vi "Configure Multicolumn Listbox for Displayed Samples.vi"(7 "Samples":i64, 8 "error in":errorcluster, 11 "MulticolumnListbox in":refnum<vi>) -> (0 "error out":errorcluster, 3 "MulticolumnListbox out":refnum<vi>)   [LabVIEW 2018, in "NI_TDMS File Viewer.lvlib"]
uses:
  NI_TDMS File Viewer.lvlib
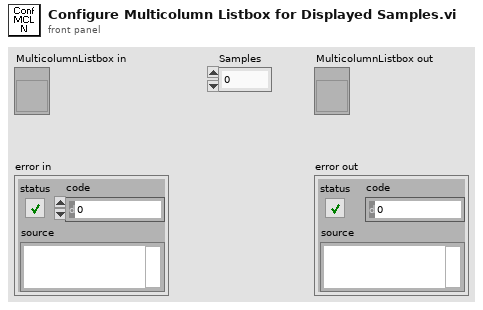
[diagram p1: front panel]
types:
  T1 = typedef "LVRowAndColumnUnsignedTypeDef.ctl" = cluster{"Row":u32, "Column":u32}
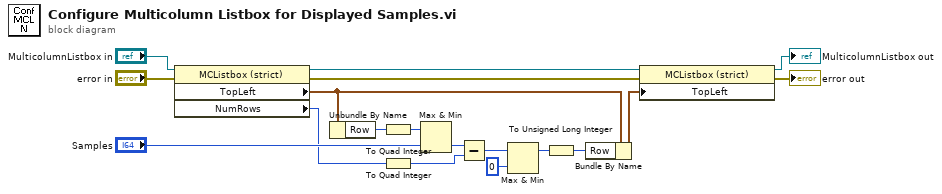
[diagram p0: block diagram]
diagram:
  n1 = property class="MCListbox (strict)"(reference="MulticolumnListbox in", error in="error in") -> (reference out=w4:refnum<vi>, error out=w17:errorcluster, "TopLeft"=w5:T1, "NumRows"=w11:u32)
  n2 = Unbundle By Name(w5) -> ("Row"=w3:u32)
  n3 = To Quad Integer(1:w3) -> (0:w13:i64)
  n4 = To Quad Integer(1:w11) -> (0:w14:i64)
  n5 = Max & Min(x=w13, y="Samples") -> (min(x,y)=w9:i64)  [unwired: 1 out]
  n6 = Subtract(x=w9, y=w14) -> (x-y=w7:i64)
  n7 = Max & Min(x=w7, y=i64 0) -> (max(x,y)=w10:i64)  [unwired: 1 out]
  n8 = To Unsigned Long Integer(number=w10) -> (unsigned 32bit integer=w15:u32)
  n9 = Bundle By Name(cluster=w5, "Row"=w15) -> (w6:T1)
  n10 = property class="MCListbox (strict)"(reference=w4, error in=w17, "TopLeft"=w6) -> (reference out=→"MulticolumnListbox out":refnum<vi>, error out=→"error out":errorcluster)
